vi "Read Sub Panel Coin.vi"(8 "error in (no error)":errorcluster, 11 "Monedas MXN in":refnum<class "Monedas MXN.lvclass">) -> (0 "error out":errorcluster, 2 "Sub Panel Coin":refnum<vi>, 3 "Monedas MXN out":refnum<class "Monedas MXN.lvclass">)   [LabVIEW 2020, in "Monedas MXN.lvlib" / "Monedas MXN.lvclass"]
uses:
  Monedas MXN.lvclass
  Monedas MXN.lvclass/Monedas MXN.ctl
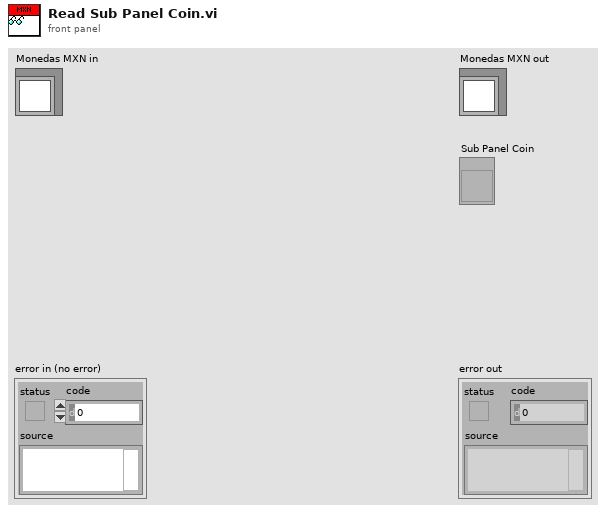
[diagram p1: front panel]
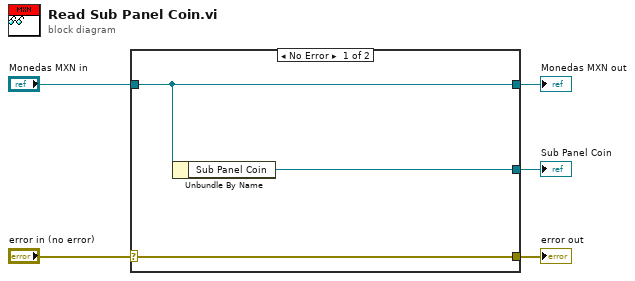
[diagram p0: block diagram]
diagram:
  n1 = case shown="No Error" "error in (no error)" {
    selector: "error in (no error)" -> [w8 w9]
    tunnel: [w8 w9] -> w4
    tunnel: [w7 w10] -> w2
    tunnel: "Monedas MXN in" -> [w7 w10]
    tunnel: [w6 _] -> w1
    frame No Error {
      n2 = Unbundle By Name(w7) -> ("Sub Panel Coin"=w6:refnum<vi>)
    }
    frame Error {
    }
  }
  "error out" <- w4
  "Monedas MXN out" <- w2
  "Sub Panel Coin" <- w1
